vi "sv_UFF58 Write Abscissa (Record 7).vi"(0 "function refnum":refnum<k20>, 1 "data precision (double-precision:1)":T1=1 items=["single-precision", "double-precision"], 5 "Name":string="Time", 7 "x0":dbl, 9 "dx":dbl, 11 "error in (no error)":errorcluster, 12 "channel length":i32) -> (4 "dup function refnum":refnum<k20>, 15 "error out":errorcluster)   [LabVIEW 2017, in "SoundVib_UFF58.lvlib"]
doc: "This VI writes <B>x0</B> and <B>dx</B> values for the record 7 fields 4 and 5 respectively"
uses:
  <vilib>/addons/Sound and Vibration/svt_UFF58/SoundVib_UFF58.lvlib
  <vilib>/addons/Sound and Vibration/svt_UFF58/subVIs/sv_UFF58 Data Precision.ctl
  <vilib>/Platform/storage/Storage.llb/Set Property (I32).vi
  <vilib>/Platform/storage/Storage.llb/Get Property (Storage Refnums).vi
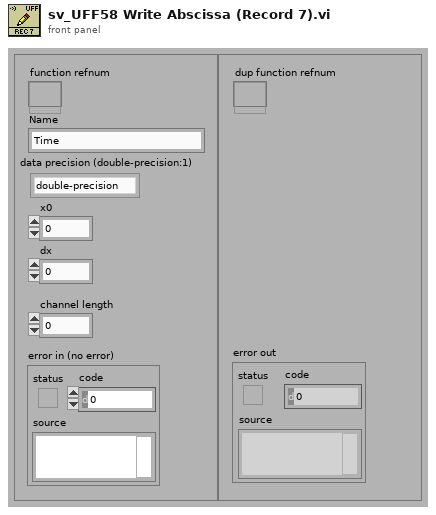
[diagram p1: front panel]
types:
  T1 = typedef "SoundVib_UFF58.lvlib/sv_UFF58 Data Precision.ctl" = u32
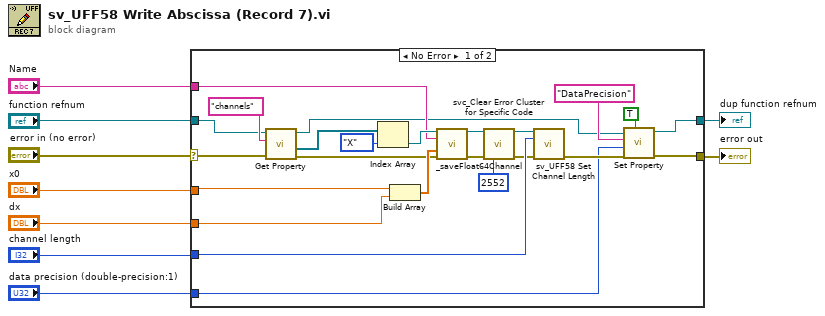
[diagram p0: block diagram]
diagram:
  n1 = case shown="No Error" "error in (no error)" {
    selector: "error in (no error)" -> [w26 w33]
    tunnel: [w14 w33] -> w9
    tunnel: "function refnum" -> [w28 w34]
    tunnel: [w12 w34] -> w2
    tunnel: "x0" -> [w25 _]
    tunnel: "dx" -> [w24 _]
    tunnel: "Name" -> [w23 _]
    tunnel: "channel length" -> [w21 _]
    tunnel: "data precision (double-precision:1)" -> [w10 _]
    frame No Error {
      n2 = call-poly <vilib>:"Get Property.vi"("error in (no error)"=w26, "Property name"="channels", "storage refnum"=w28) -> ("error out"=w27:errorcluster, "Value"=w31:refnum<k20>[], "storage refnum out"=w13:refnum<k20>)  [unwired: 6 in]
      n3 = Index Array(array=w31, index=enum16{"X", "Y Real", "Y Imaginary"}."X" ("channel to write")) -> (element=w29:refnum<k20>)
      n4 = Build Array(w25, w24) -> (w32:dbl[])
      n5 = call <vilib>:"_saveFloat64Channel.vi"("Data object in"=w29, "Name"=w23, "Values"=w32, "error in (no error)"=w27) -> ("Data object out"=w22:refnum<k20>, "error out"=w19:errorcluster)  [unwired: 9 in, 1 out]
      n6 = call <vilib>:"svc_Clear Error Cluster for Specific Code.vi"("error in (no error)"=w19, "code"=2552 ("warning code")) -> ("error out"=w18:errorcluster)  [unwired: 12 in, 1 out]
      n7 = call <vilib>:"sv_UFF58 Set Channel Length.vi"("channel refnum"=w22, "channel length"=w21, "error in"=w18) -> ("error out"=w15:errorcluster)  [unwired: 11 in, 1 out]
      n8 = call-poly <vilib>:"Set Property.vi"("Create if not found (no:F)"=TRUE, "error in (no error)"=w15, "Value"=w10, "Property name"="DataPrecision" ("property name"), "storage refnum"=w13) -> ("error out"=w14:errorcluster, "storage refnum out"=w12:refnum<k20>)  [unwired: 5 in]
    }
    frame Error {
    }
  }
  "error out" <- w9
  "dup function refnum" <- w2
